vi "ADAM_scan_table.vi"() -> ()   [LabVIEW 2010]
uses:
  Anemometry/Anemometry Sub Vis/Controls/Serveds.ctl
  ADAM Client/Sub VIs/ADAM Controls/Module_type_ADAM.ctl
  ADAM Client/Sub VIs/ADAM Controls/Traverse_Level_State.ctl
  Anemometry/Anemometry Sub Vis/Controls/Post_Process.ctl
  ADAM Client/Sub VIs/ADAM Controls/Channel_State.ctl
  ADAM Client/Sub VIs/ADAM Controls/Ch_description_ADAM.ctl
  ADAM Client/Sub VIs/ADAM Controls/Function_ADAM.ctl
  ADAM Client/Sub VIs/ADAM Controls/Calib_type_ADAM.ctl
  ADAM Client/Sub VIs/ADAM Controls/Address.ctl
  ADAM_Global.vi
  Sub VI's/Channel_Description_Global.vi
  Anemometry/Anemometry Sub Vis/Globals/Meas_global.vi
  Sub VI's/Logged_Data_real_Global.vi
  Anemometry/Anemometry Sub Vis/Globals/Preference_global.vi
  Anemometry/Anemometry Sub Vis/Globals/Gas_management_global.vi
  Anemometry/Anemometry Sub Vis/Globals/Constants_global.vi
panel:
  in  "Reconfigure Gills":bool
  in  "Full Res Pathname":path
  in  "Log full Res Data":bool
  out "Duty No":u16 format="%.0b"
  in  "Save Current setup":bool=TRUE
  in  "Load setup from file":bool
  out "ADAM scan comments":string
  out "History length":i32=250
  in  "stop":bool
  out "Results":dbl[](array[numeric]) format="%.3f"
  out "Titles":string[](array[string])
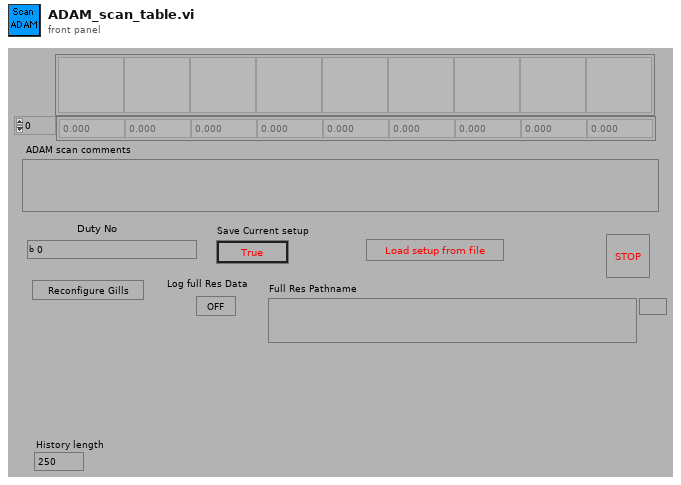
[diagram p1: front panel]
types:
  T1 = enum16{"Load ADAM setup from excel file", "Save ADAM setup to excel file"}
  T2 = typedef "Serveds.ctl" = enum16{"Read Global", "Load Global From File"}
  T3 = typedef "Module_type_ADAM.ctl" = enum16{"4011", "4012", "4013", "4014", "4016", "4017", "4018", "4021", "4050", "4052", "4053", "4060", "4080", "5000", "5017", "5018", "5024", "5051", "5056", "5060", "6060", "Tracker", "WEST", "GILL", "JEM", "VICI", "Vaisala", "DRUCK", "Run VI Named:", "IR2100", "PPT", "Comparator", "VIRTUAL", "Hold Value", "Read A", "Read Ch", "Coded", "Client Info", "Web Client", "X10", "Test"}
  T4 = typedef "Traverse_Level_State.ctl" = enum16{"Running", "Complete"}
  T5 = typedef "Post_Process.ctl" = enum16{"Take New Data", "Post Process Raw Data File"}
  T6 = typedef "Channel_State.ctl" = enum16{"On", "Off", "Always On", "Always Off"}
  T7 = enum16{"Append to Global", "Read Global then Clear"}
  T8 = typedef "Ch_description_ADAM.ctl" = cluster{"Ch Name":string, "Type":T3, "Function":T9, "Ch State":T6, "Calibration type":T10, "A":dbl, "B":dbl, "C":dbl, "D":dbl, "Comments":string, "Address":T11, "String":string, "Duty":u16}
  T9 = typedef "Function_ADAM.ctl" = enum16{"Analogue Input", "Digital Input", "Event counter", "Event rate", "Analogue Output", "Digital Output", "Relay Output"}
  T10 = typedef "Calib_type_ADAM.ctl" = enum16{"Raw", "Bx + A", "Cx^2 + Bx + A", "Dx^3 + Cx^2 + Bx + A", "In Band", "Hi-Tec Q", "Hi-Tec M_dot", "Text"}
  T11 = typedef "Address.ctl" = cluster{"Main":i32, "Ch.":i32, "Sub":i32, "Port Name":string}
  T12 = typedef "Client_State_Cluster.ctl" = cluster{"Client Name":string, "Traverse level State":T4, "People to Email":string[], "Next Contact Time":dbl}
  T13 = typedef "Update_scan_value.ctl" = cluster{"Channel Name":string, "New Value":dbl}
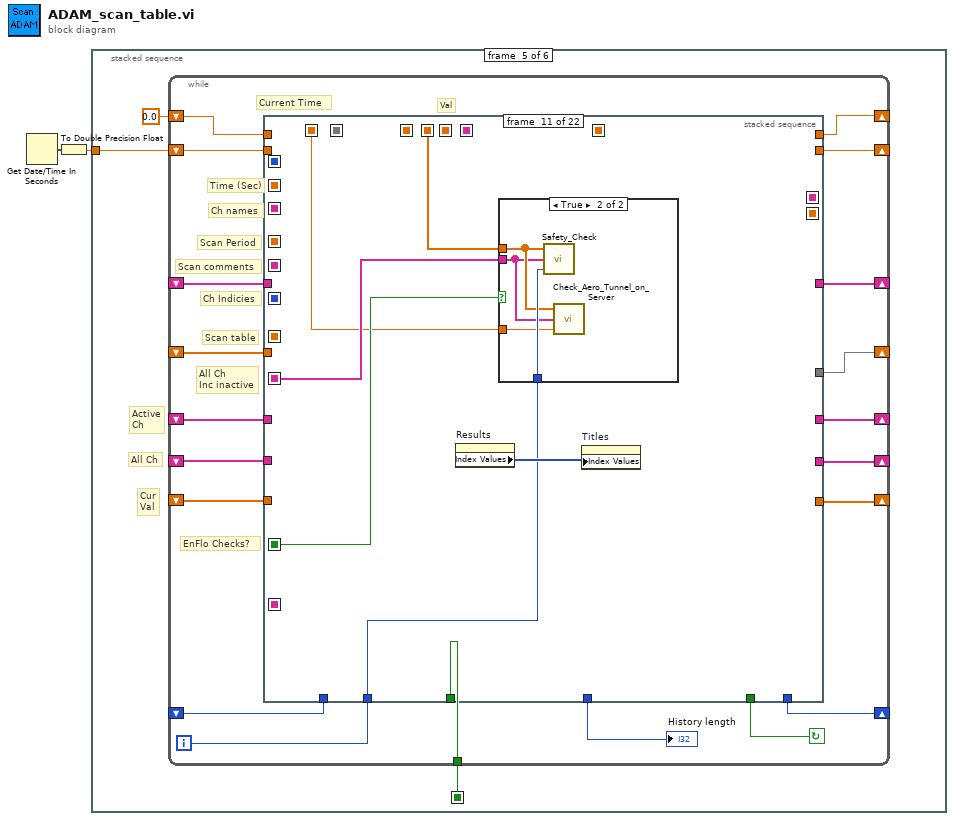
[diagram p0: block diagram]
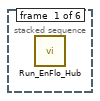
[diagram p2: hidden frame]
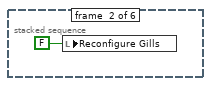
[diagram p3: hidden frame]
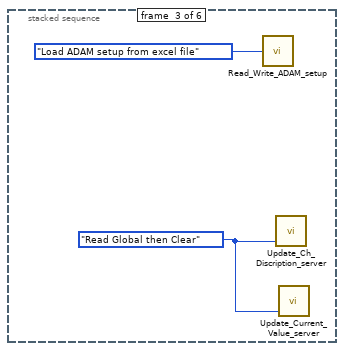
[diagram p4: hidden frame]
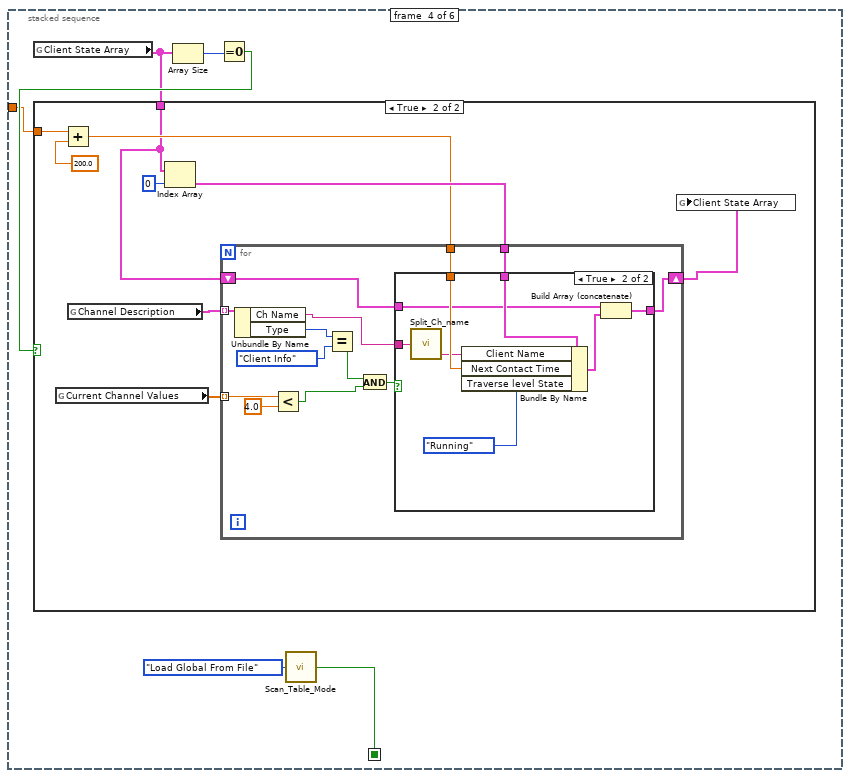
[diagram p5: hidden frame]
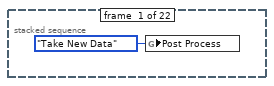
[diagram p8: hidden frame]
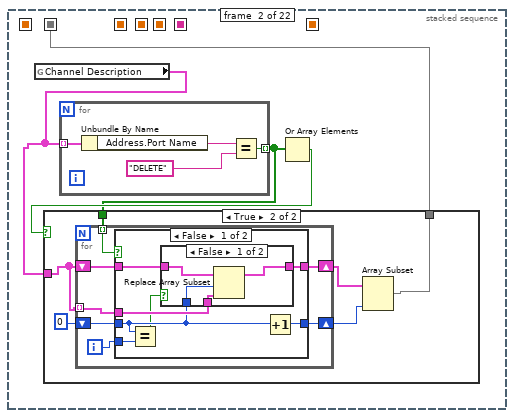
[diagram p9: hidden frame]
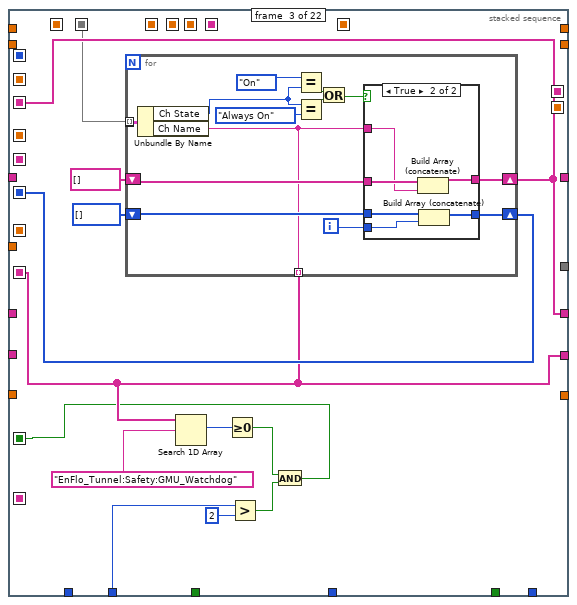
[diagram p13: hidden frame]
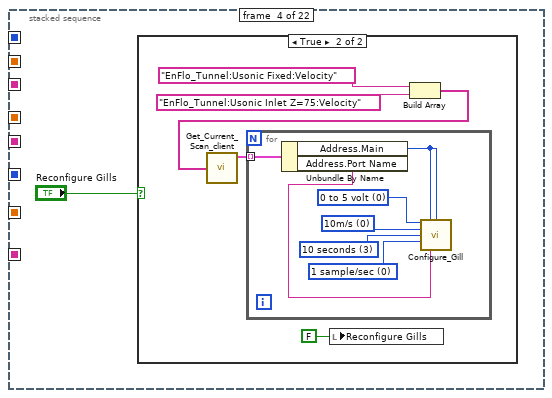
[diagram p15: hidden frame]
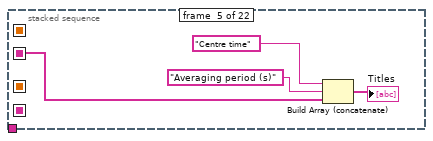
[diagram p17: hidden frame]
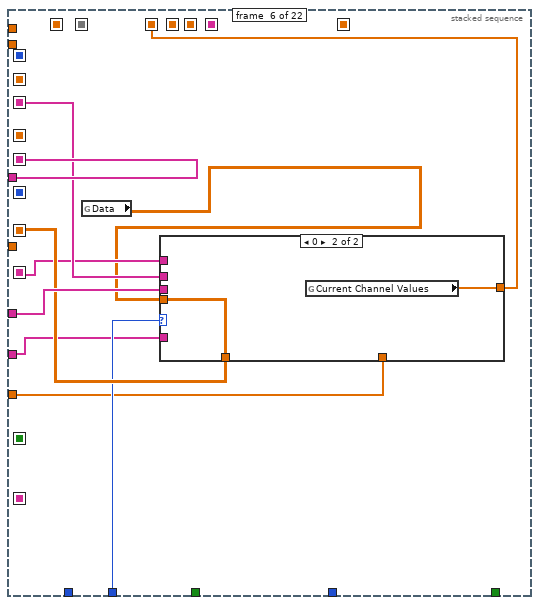
[diagram p18: hidden frame]
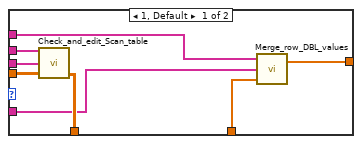
[diagram p19: hidden frame]
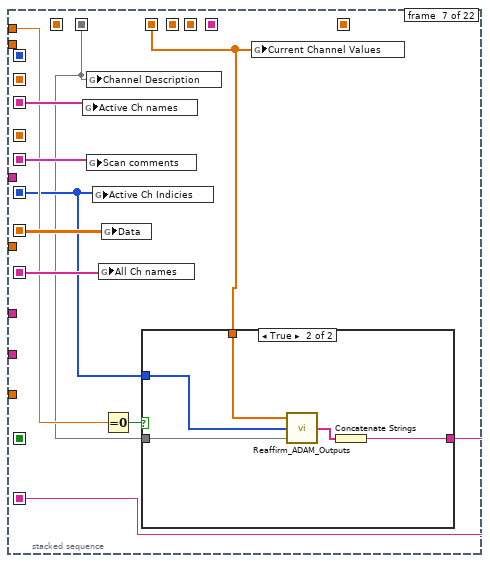
[diagram p20: hidden frame]
diagram:
  n1 = Get Date/Time In Seconds() -> (seconds since 1Jan1904=w2:timestamp)
  n2 = To Double Precision Float(number=w2) -> (double precision float=w1:dbl)
  n3 = stacked-sequence {
    seq-local: [_ _ _ w11 _ _] -> [_ _ _ _ w45 _]
    tunnel: w1 -> [_ _ _ w6 w43 _]
    frame #0 {
      n4 = call "Run_EnFlo_Hub.vi"() -> ()  [unwired: 8 out]
    }
    frame #1 {
      n5 = local write "Reconfigure Gills"(FALSE ("Reconfigure Gills")) -> ()
    }
    frame #2 {
      w4 = T7."Read Global then Clear" ("Mode")
      n6 = call "Read_Write_ADAM_setup.vi"("Mode"=T1."Load ADAM setup from excel file") -> ()  [unwired: 4 out]
      n7 = call "Update_Ch_Discription_server.vi"("Mode"=w4) -> ()  [unwired: 2 in, 1 out]
      n8 = call "Update_Current_Value_server.vi"("Mode"=w4) -> ()  [unwired: 2 in, 1 out]
    }
    frame #3 {
      n9 = global read "ADAM_Global.vi" "Client State Array"() -> (w7:T12[])
      n10 = Array Size(array=w7) -> (size(s)=w9:i32)
      n11 = Equal To 0?(x=w9) -> (x = 0?=w8:bool)
      n12 = case shown="True" w8 {
        tunnel: w7 -> [_ w13]
        tunnel: w6 -> [_ w16]
        frame False {
        }
        frame True {
          n13 = global read "ADAM_Global.vi" "Current Channel Values"() -> (w20:dbl[])
          n14 = Add(x=w16, y=200.0) -> (x+y=w14:dbl)
          n15 = global read "Channel_Description_Global.vi" "Channel Description"() -> (w19:T8[])
          n16 = Index Array(array=w13, index=0) -> (element=w17:T12)
          n17 = for {
            tunnel: w19 -> [w33] mode=indexing
            tunnel: w20 -> [w25] mode=indexing
            tunnel: w17 -> [w26]
            tunnel: w14 -> [w24]
            shift-right: [w23] -> w12
            shift-left: w13 -> [w22]
            n18 = Unbundle By Name(w33) -> ("Ch Name"=w21:string, "Type"=w30:T3)
            n19 = Less?(x=w25, y=4.0) -> (x < y?=w28:bool)
            n20 = Equal?(x=w30, y=Module_type_ADAM."Client Info" ("Type")) -> (x = y?=w29:bool)
            n21 = And(x=w29, y=w28) -> (x .and. y?=w27:bool)
            n22 = case shown="True" w27 {
              tunnel: w26 -> [_ w42]
              tunnel: w24 -> [_ w41]
              tunnel: [w34 w39] -> w23
              tunnel: w22 -> [w34 w38]
              tunnel: w21 -> [_ w36]
              frame False {
              }
              frame True {
                n23 = call "Split_Ch_name.vi"("Ch name"=w36) -> ("Low level"=w35:string)  [unwired: 2 out]
                n24 = Bundle By Name(cluster=w42, "Client Name"=w35, "Next Contact Time"=w41, "Traverse level State"=Traverse_Level_State."Running") -> (w37:T12)
                n25 = Build Array (concatenate)(w38, w37) -> (w39:T12[])
              }
            }
          }
          n26 = global write "ADAM_Global.vi" "Client State Array"(w12) -> ()
        }
      }
      n27 = call "Scan_Table_Mode.vi"("Mode"=Serveds."Load Global From File") -> ("Simulate Mode ?"=w11:bool)
    }
    frame #4 {
      # "Active\nCh"
      # "Cur\nVal"
      # "All Ch"
      n28 = while {
        shift-left: _ -> [w47]
        shift-right: [w46] -> _
        shift-left: _ -> [w48]
        shift-right: [w49] -> _
        shift-left: _ -> [w50]
        shift-right: [w51] -> _
        tunnel: w45 -> [w53]
        shift-left: _ -> [w56]
        shift-right: [w55] -> _
        shift-left: 0.0 -> [w57]
        shift-right: [w52] -> _
        shift-left: _ -> [w59]
        shift-right: [w60] -> _
        shift-left: _ -> [w61]
        shift-right: [w62] -> _
        shift-left: w43 -> [w63]
        shift-right: [w64] -> _
        i -> [w58]
        stop <- w65 continue-if-true
        # "Current Time"
        # "EnFlo Checks?"
        # "Val"
        # "All Ch\nInc inactive"
        # "Scan comments"
        # "Scan table"
        # "Time (Sec)"
        # "Ch Indicies"
        # "Ch names"
        # "Scan Period"
        n29 = stacked-sequence {
          seq-local: [_ _ _ _ _ _ _ _ _ _ _ _ w282 _ _ _ _ _ _ _ _ _] -> [_ _ _ _ _ _ _ _ _ _ _ _ _ _ w333 w338 _ _ _ _ w416 _]
          seq-local: [_ _ _ _ _ _ _ w193 _ _ _ _ _ _ _ _ _ _ _ _ _ _] -> [_ _ _ _ _ _ _ _ _ _ _ _ _ _ _ w345 _ _ _ _ _ _]
          seq-local: [_ _ _ _ _ w160 _ _ _ _ _ _ _ _ _ _ _ _ _ _ _ _] -> [_ _ _ _ _ _ w180 _ _ _ _ _ _ _ _ w343 _ _ _ _ _ _]
          seq-local: [_ _ _ _ _ _ _ w197 _ _ _ _ _ _ _ _ _ _ _ _ _ _] -> [_ _ _ _ _ _ _ _ _ w220 _ w249 _ _ _ w344 _ _ _ _ _ _]
          seq-local: [_ _ _ _ _ w163 _ _ _ _ _ _ _ _ _ _ _ _ _ _ _ _] -> [_ _ _ _ _ _ w182 _ _ _ _ _ _ _ _ _ _ w383 _ _ _ _]
          seq-local: [_ _ _ _ _ _ _ _ _ w218 _ _ _ _ _ _ _ _ _ _ _ _] -> [_ _ _ _ _ _ _ _ _ _ _ _ _ _ _ _ _ w371 _ _ _ _]
          seq-local: [_ _ w114 _ _ _ _ _ _ _ _ _ _ _ _ _ _ _ _ _ _ _] -> [_ _ _ _ w152 w162 w183 w198 _ _ _ _ _ _ _ w341 w346 _ _ _ _ _]
          seq-local: [_ _ w113 _ _ _ _ _ _ _ _ _ _ _ _ _ _ _ _ _ _ _] -> [_ _ _ _ _ _ w176 _ _ w219 _ _ _ _ _ _ _ _ _ _ _ _]
          seq-local: [_ _ _ _ _ w156 _ _ _ _ _ _ _ _ _ _ _ _ _ _ _ _] -> [_ _ _ _ _ _ w177 _ _ w216 _ _ _ _ _ _ _ _ _ _ _ _]
          seq-local: [_ _ _ _ _ _ _ _ _ w214 _ _ _ _ _ _ _ _ _ _ _ _] -> [_ _ _ _ _ _ _ _ _ _ w240 w248 w280 _ _ _ _ _ _ _ _ _]
          seq-local: [_ _ w109 _ _ _ _ _ _ _ _ _ _ _ _ _ _ _ _ _ _ _] -> [_ _ _ _ _ w158 w181 _ _ w215 w239 w247 w281 w306 w325 w340 _ _ _ w393 _ _]
          seq-local: [_ _ _ _ _ _ _ _ w200 _ _ _ _ _ _ _ _ _ _ _ _ _] -> [_ _ _ _ _ _ _ _ _ w213 _ _ _ _ _ _ _ _ _ _ _ _]
          seq-local: [_ w67 _ _ _ _ _ _ _ _ _ _ _ _ _ _ _ _ _ _ _ _] -> [_ _ w111 _ _ _ w175 _ _ w212 _ _ _ _ _ _ _ _ _ _ _ _]
          seq-local: [_ _ _ _ _ _ _ w192 _ _ _ _ _ _ _ _ _ _ _ _ _ _] -> [_ _ _ _ _ _ _ _ _ _ w236 _ _ _ _ _ w348 _ _ _ _ _]
          seq-local: [_ _ _ _ _ _ _ _ _ _ _ _ _ _ _ w337 _ _ _ _ _ _] -> [_ _ _ _ _ _ _ _ _ _ _ _ _ _ _ _ w347 _ _ _ _ _]
          seq-local: [_ _ w103 _ _ _ _ _ _ _ _ _ _ _ _ _ _ _ _ _ _ _] -> [_ _ _ _ _ _ _ w190 _ _ w238 w246 _ _ _ _ _ _ _ _ _ _]
          seq-local: [_ _ _ _ _ _ _ _ _ _ _ _ w279 _ _ _ _ _ _ _ _ _] -> [_ _ _ _ _ _ _ _ _ _ _ _ _ w307 _ _ _ _ _ _ _ _]
          seq-local: [_ _ _ _ _ _ w174 _ _ _ _ _ _ _ _ _ _ _ _ _ _ _] -> [_ _ _ _ _ _ _ _ _ w211 _ _ _ _ _ _ _ _ _ _ _ _]
          seq-local: [_ _ _ _ _ _ _ _ _ _ _ _ w278 _ _ _ _ _ _ _ _ _] -> [_ _ _ _ _ _ _ _ _ _ _ _ _ w305 _ _ _ _ _ _ _ _]
          tunnel: [_ _ _ _ _ _ _ _ _ _ _ _ _ _ _ _ _ _ w391 _ _ _] -> w65
          tunnel: [_ _ _ _ _ _ _ w192 _ _ _ _ _ _ _ _ _ _ _ _ _ _] -> w64
          tunnel: w63 -> [_ _ _ _ _ _ _ w194 _ _ _ _ _ _ _ _ _ _ _ _ _ _]
          tunnel: [_ _ _ _ _ _ _ _ _ _ _ _ _ _ _ _ _ w381 _ _ _ _] -> w62
          tunnel: w61 -> [_ _ _ _ _ w163 _ _ _ _ _ _ _ _ _ _ _ _ _ _ _ _]
          tunnel: [_ _ w114 _ _ _ _ _ _ _ _ _ _ _ _ _ _ _ _ _ _ _] -> w60
          tunnel: w59 -> [_ _ _ _ _ w161 _ _ _ _ _ _ _ w308 _ _ _ _ _ _ _ _]
          tunnel: w58 -> [_ _ w107 _ _ w159 _ _ _ _ w237 _ _ _ _ _ _ _ w389 _ _ w420]
          tunnel: w57 -> [_ _ _ _ _ _ w178 _ _ _ _ w251 _ _ _ _ _ _ _ _ _ _]
          tunnel: [_ _ _ _ _ _ _ _ _ _ _ w253 _ _ _ _ _ _ _ _ _ _] -> w52
          tunnel: w56 -> [_ _ _ _ _ _ _ _ _ _ _ _ _ _ w331 _ _ _ _ _ _ _]
          tunnel: [_ _ _ _ _ _ _ _ _ _ _ _ _ _ w327 _ _ _ _ _ _ _] -> w55
          tunnel: [_ _ _ _ _ _ _ _ _ _ _ _ _ _ _ w342 _ _ _ _ _ _] -> w54
          tunnel: w53 -> [_ _ _ _ _ _ _ _ _ w217 _ _ _ _ _ _ _ _ _ _ _ _]
          tunnel: [_ _ w109 _ _ _ _ _ _ _ _ _ _ _ _ _ _ _ _ _ _ _] -> w51
          tunnel: w50 -> [_ _ _ _ _ w157 _ _ _ _ _ _ _ _ _ _ _ _ _ _ _ _]
          tunnel: [_ _ _ _ _ _ _ _ _ _ _ _ _ _ _ _ _ _ _ _ w416 _] -> w49
          tunnel: w48 -> [_ _ _ _ _ w155 _ _ _ _ _ _ _ _ _ _ _ _ _ _ _ _]
          tunnel: w47 -> [_ _ _ _ _ _ _ _ w201 _ _ _ _ _ _ _ _ _ _ _ _ _]
          tunnel: [_ _ _ _ _ _ _ _ w202 _ _ _ _ _ _ _ _ _ _ _ _ _] -> w46
          frame #0 {
            n30 = global write "Meas_global.vi" "Post Process"(Post_Process."Take New Data" ("Post Process")) -> ()
          }
          frame #1 {
            n31 = global read "Channel_Description_Global.vi" "Channel Description"() -> (w69:T8[])
            n32 = for {
              tunnel: w69 -> [w102] mode=indexing
              tunnel: [w99] -> w68 mode=indexing
              n33 = Unbundle By Name(w102) -> ("Address.Port Name"=w101:string)
              n34 = Equal?(x=w101, y="DELETE") -> (x = y?=w99:bool)
            }
            n35 = Or Array Elements(Boolean array=w68) -> (logical OR=w70:bool)
            n36 = case shown="True" w70 {
              tunnel: w69 -> [w71 w75]
              tunnel: w68 -> [_ w77]
              tunnel: [w71 w72] -> w67
              frame False {
              }
              frame True {
                n37 = for {
                  shift-right: [w84] -> w74
                  shift-left: w75 -> [w83]
                  tunnel: w77 -> [w79] mode=indexing
                  shift-right: [w82] -> w73
                  shift-left: 0 -> [w80]
                  tunnel: w75 -> [w81] mode=indexing
                  i -> [w78]
                  n38 = case shown="False" w79 {
                    tunnel: [w90 w98] -> w84
                    tunnel: w83 -> [w91 w98]
                    tunnel: [w88 w97] -> w82
                    tunnel: w80 -> [w87 w97]
                    tunnel: w81 -> [w89 _]
                    tunnel: w78 -> [w86 _]
                    frame False {
                      n39 = Equal?(x=w87, y=w86) -> (x = y?=w85:bool)
                      n40 = case shown="False" w85 {
                        tunnel: w91 -> [w95 w96]
                        tunnel: [w94 w96] -> w90
                        tunnel: w89 -> [w93 _]
                        tunnel: w87 -> [w92 _]
                        frame False {
                          n41 = Replace Array Subset(array=w95, new element=w93, index=w92) -> (w94:T8[])
                        }
                        frame True {
                        }
                      }
                      n42 = Increment(x=w87) -> (x+1=w88:i32)
                    }
                    frame True {
                    }
                  }
                }
                n43 = Array Subset(array=w74, length=w73) -> (w72:T8[])  [unwired: 1 in]
              }
            }
          }
          frame #2 {
            n44 = for {
              tunnel: [w128] -> _ mode=indexing
              shift-right: [w127] -> w114
              shift-left: string[] [] -> [w118]
              shift-right: [w124] -> w113
              shift-left: i32[] [] -> [w126]
              tunnel: [w116] -> w109 mode=indexing
              tunnel: w111 -> [w128] mode=indexing
              i -> [w125]
              n45 = Unbundle By Name(w128) -> ("Ch State"=w119:T6, "Ch Name"=w116:string)
              n46 = Equal?(x=Channel_State."On" ("Channel State"), y=w119) -> (x = y?=w121:bool)
              n47 = Equal?(x=w119, y=Channel_State."Always On" ("Channel State")) -> (x = y?=w120:bool)
              n48 = Or(x=w121, y=w120) -> (x .or. y?=w117:bool)
              n49 = case shown="True" w117 {
                tunnel: w118 -> [w129 w136]
                tunnel: w116 -> [_ w135]
                tunnel: [w129 w134] -> w127
                tunnel: w126 -> [w130 w133]
                tunnel: w125 -> [_ w132]
                tunnel: [w130 w131] -> w124
                frame False {
                }
                frame True {
                  n50 = Build Array (concatenate)(w136, w135) -> (w134:string[])
                  n51 = Build Array (concatenate)(w133, w132) -> (w131:i32[])
                }
              }
            }
            n52 = Search 1D Array(1D array=w109, element="EnFlo_Tunnel:Safety:GMU_Watchdog") -> (index of element=w108:i32)  [unwired: 1 out]
            n53 = Greater Or Equal To 0?(x=w108) -> (x >= 0?=w104:bool)
            n54 = Greater?(x=w107, y=2) -> (0:w105:bool)
            n55 = And(x=w104, y=w105) -> (x .and. y?=w103:bool)
          }
          frame #3 {
            n56 = case shown="True" "Reconfigure Gills" {
              frame False {
              }
              frame True {
                n57 = local write "Reconfigure Gills"(FALSE ("Reconfigure Gills")) -> ()
                n58 = Build Array("EnFlo_Tunnel:Usonic Fixed:Velocity", "EnFlo_Tunnel:Usonic Inlet Z=75:Velocity") -> (w140:string[])
                n59 = call "Get_Current_Scan_client.vi"("ADAM Ch Names"=w140) -> ("Ch Description Array"=w139:T8[])  [unwired: 3 out]
                n60 = for {
                  tunnel: w139 -> [w145] mode=indexing
                  w149 = u16 0 items=["1 sample/sec", "4 samples/sec"] ("Samples/sec")
                  w148 = u16 3 items=["OFF", "3 seconds", "5 seconds", "10 seconds"] ("Averaging Time")
                  w147 = u16 0 items=["10m/s", "20m/s", "30m/s", "40m/s", "50m/s", "60m/s", "70m/s"] ("Analogue O/P Scale")
                  w146 = u16 0 items=["0 to 5 volt", "+/-2.5 Volt", "4-20mA"] ("Analogue O/P Config")
                  n61 = Unbundle By Name(w145) -> ("Address.Main"=w144:i32, "Address.Port Name"=w143:string)
                  n62 = call "Configure_Gill.vi"("Analogue O/P Config"=w146, "ORIGINAL Address"=w144, "NEW Address"=w144, "Analogue O/P Scale"=w147, "Averaging Time"=w148, "Samples/sec"=w149, "Port Name"=w143) -> ()  [unwired: 9 out]
                }
              }
            }
          }
          frame #4 {
            n63 = Build Array (concatenate)("Centre time", "Averaging period (s)", w152) -> (→"Titles":string[])
          }
          frame #5 {
            n64 = global read "Logged_Data_real_Global.vi" "Data"() -> (w154:dbl[][])
            n65 = case shown="0" w159 {
              tunnel: w154 -> [w171 w173]
              tunnel: w162 -> [w168 _]
              tunnel: w161 -> [w170 _]
              tunnel: [w169 w173] -> w160
              tunnel: w158 -> [w167 _]
              tunnel: w157 -> [w166 _]
              tunnel: [w165 w172] -> w156
              tunnel: w155 -> [w164 _]
              frame 1, Default {
                n66 = call "Check_and_edit_Scan_table.vi"("2D array input"=w171, "Original Channels"=w170, "Present Channels"=w168) -> ("2D array output"=w169:dbl[][])  [unwired: 2 out]
                n67 = call "Merge_row_DBL_values.vi"("Present Row values"=w164, "Present Channels"=w166, "Desired Channels"=w167) -> ("Desired Row values"=w165:dbl[])  [unwired: 1 out]
              }
              frame 0 {
                n68 = global read "ADAM_Global.vi" "Current Channel Values"() -> (w172:dbl[])
              }
            }
          }
          frame #6 {
            n69 = global write "ADAM_Global.vi" "Active Ch names"(w183) -> ()
            n70 = global write "Channel_Description_Global.vi" "Channel Description"(w175) -> ()
            n71 = global write "ADAM_Global.vi" "Scan comments"(w182) -> ()
            n72 = global write "ADAM_Global.vi" "Active Ch Indicies"(w176) -> ()
            n73 = global write "ADAM_Global.vi" "All Ch names"(w181) -> ()
            n74 = global write "Logged_Data_real_Global.vi" "Data"(w180) -> ()
            n75 = Equal To 0?(x=w178) -> (x = 0?=w179:bool)
            n76 = case shown="True" w179 {
              tunnel: w177 -> [_ w189]
              tunnel: w176 -> [_ w188]
              tunnel: w175 -> [_ w187]
              tunnel: ["" w185] -> w174
              frame False {
              }
              frame True {
                n77 = call "Reaffirm_ADAM_Outputs.vi"("Channel Description"=w187, "Active Ch Indicies"=w188, "Current Channel Values"=w189) -> ("Scan Comments"=w186:string[])  [unwired: 2 out]
                n78 = Concatenate Strings(w186) -> (w185:string)
              }
            }
            n79 = global write "ADAM_Global.vi" "Current Channel Values"(w177) -> ()
          }
          frame #7 {
            n80 = case shown="True" w190 {
              tunnel: w198 -> [_ w199]
              frame False {
              }
              frame True {
                n81 = call "Gas_Status_panel.vi"("Ch names"=w199) -> ()  [unwired: 15 out]
              }
            }
            n82 = Get Date/Time In Seconds() -> (seconds since 1Jan1904=w191:timestamp)
            n83 = To Double Precision Float(number=w191) -> (double precision float=w192:dbl)
            n84 = Subtract(x=w192, y=w194) -> (x-y=w197:dbl)
            n85 = Divide(x=w197, y=2.0) -> (x/y=w195:dbl)
            n86 = Add(x=w195, y=w194) -> (x+y=w193:dbl)
          }
          frame #8 {
            n87 = Equal To 0?(x=w201) -> (x = 0?=w205:bool)
            n88 = Equal?(x=u16 32768, y=w201) -> (x = y?=w204:bool)
            n89 = Select(t=u16 1, s=w205, f=w201) -> (s? t:f=w200:u16)
            "Duty No" <- w200
            n90 = case shown="False" w204 {
              tunnel: [w207 u16 0] -> w202
              tunnel: w200 -> [w209 _]
              frame False {
                n91 = Multiply(x=u16 2, y=w209) -> (x*y=w207:u16)
              }
              frame True {
              }
            }
          }
          frame #9 {
            n92 = for {
              tunnel: w212 -> [w227]
              tunnel: w220 -> [w235]
              shift-right: [w233] -> w214
              shift-left: w216 -> [w231]
              tunnel: w215 -> [w232]
              shift-right: [w228] -> w218
              shift-left: w211 -> [w230]
              tunnel: w219 -> [w222] mode=indexing
              tunnel: w216 -> [w224]
              tunnel: w217 -> [w225]
              tunnel: w213 -> [w221]
              n93 = Index Array(array=w224, index=w222) -> (element=w223:dbl)
              n94 = Index Array(array=w227, index=w222) -> (element=w226:T8)
              n95 = call "Adam_Ch_Input_Output.vi"("Simulate"=w225, "Duty No"=w221, "Previuos Scan Value"=w223, "Ch values"=w231, "Scan Period"=w235, "Ch Discription"=w226, "Ch names"=w232) -> ("Scan comment"=w229:string, "Calibrated units"=w234:dbl)  [unwired: 1 in, 2 out]
              n96 = Concatenate Strings(w230, w229) -> (w228:string)
              n97 = Replace Array Subset(array=w231, new element=w234, index=w222) -> (w233:dbl[])
            }
          }
          frame #10 {
            n98 = property on="Results" class="Arr (strict)"() -> ("Index Values"=w241:u32[])  [unwired: 2 in, 2 out]
            n99 = case shown="True" w238 {
              tunnel: w240 -> [_ w244]
              tunnel: w239 -> [_ w243]
              tunnel: w237 -> [_ w245]
              tunnel: w236 -> [_ w242]
              frame False {
              }
              frame True {
                n100 = call "Safety_Check.vi"("Adam Loop Count"=w245, "Ch Names"=w243, "Values"=w244) -> ()  [unwired: 1 out]
                n101 = call "Check_Aero_Tunnel_on_Server.vi"("Current Time"=w242, "Ch Names"=w243, "Values"=w244) -> ()  [unwired: 1 in]
              }
            }
            n102 = property on="Titles" class="Arr (strict)"("Index Values"=w241) -> ()  [unwired: 2 in, 2 out]
          }
          frame #11 {
            n103 = Greater?(x=w251, y=60.0) -> (0:w252:bool)
            n104 = case shown="True" w252 {
              tunnel: [w255 w260] -> w253
              tunnel: w251 -> [w256 _]
              tunnel: w249 -> [w254 _]
              tunnel: w248 -> [_ w259]
              tunnel: w247 -> [_ w258]
              tunnel: w246 -> [_ w257]
              frame False {
                n105 = Add(x=w256, y=w254) -> (x+y=w255:dbl)
              }
              frame True {
                n106 = stacked-sequence {
                  tunnel: [0.0 _] -> w260
                  tunnel: w259 -> [_ w275]
                  tunnel: w258 -> [_ w274]
                  tunnel: w257 -> [_ w273]
                  frame #0 {
                    n107 = case shown="False" "Save Current setup" {
                      tunnel: [FALSE w265] -> w261
                      frame False {
                      }
                      frame True {
                        n108 = Get Date/Time In Seconds() -> (seconds since 1Jan1904=w267:timestamp)
                        n109 = global read "ADAM_Global.vi" "Network Last checked"() -> (w271:dbl)
                        n110 = To Double Precision Float(number=w267) -> (double precision float=w266:dbl)
                        n111 = Subtract(x=w271, y=w266) -> (x-y=w270:dbl)
                        n112 = Absolute Value(x=w270) -> (abs(x)=w269:dbl)
                        n113 = Less?(x=w269, y=1.5) -> (x < y?=w265:bool)
                      }
                    }
                    n114 = case shown="True" w261 {
                      frame False {
                      }
                      frame True {
                        n115 = call "Read_Write_ADAM_setup.vi"("Mode"=T1."Save ADAM setup to excel file") -> ()  [unwired: 4 out]
                      }
                    }
                  }
                  frame #1 {
                    n116 = case shown="True" w273 {
                      tunnel: w275 -> [_ w277]
                      tunnel: w274 -> [_ w276]
                      frame False {
                      }
                      frame True {
                        n117 = call "Do_Every_minute.vi"("Ch Names"=w276, "Values"=w277) -> ()  [unwired: 1 out]
                      }
                    }
                  }
                }
              }
            }
          }
          frame #12 {
            n118 = call "Update_Current_Value_server.vi"("Mode"=T7."Read Global then Clear") -> ("Update array out"=w284:T13[])  [unwired: 2 in]
            n119 = for {
              tunnel: w281 -> [w292]
              tunnel: w284 -> [w287] mode=indexing
              shift-right: [w290] -> w282
              shift-left: w280 -> [w291]
              tunnel: [w286] -> w279 mode=indexing
              tunnel: [w285] -> w278 mode=indexing
              n120 = Unbundle By Name(w287) -> ("Channel Name"=w286:string, "New Value"=w285:dbl)
              n121 = Search 1D Array(1D array=w292, element=w286) -> (index of element=w289:i32)  [unwired: 1 out]
              n122 = Less Than 0?(x=w289) -> (x < 0?=w288:bool)
              n123 = case shown="True" w288 {
                tunnel: w286 -> [_ w293]
                tunnel: w287 -> [_ w298]
                frame False {
                }
                frame True {
                  n124 = global read "ADAM_Global.vi" "Update Current Value"() -> (w297:T13[])
                  n125 = call "Check_Ch_Name_colons.vi"("No of Colons"=2, "Ch Name in"=w293) -> ("Ch Name out"=w294:string)
                  n126 = Bundle By Name(cluster=T8 {"Ch Name"="", "Type"=enum."Hold Value", "Function"=enum."Analogue Input", "Ch State"=enum."On", "Calibration type"=enum."Raw", "A"=0.0, "B"=0.0, "C"=0.0, "D"=0.0, "Comments"="", "Address"={"Main"=0, "Ch."=0, "Sub"=0, "Port Name"=""}, "String"="", "Duty"=65535} ("Ch Description"), "Ch Name"=w294, "Type"=Module_type_ADAM."Hold Value") -> (w302:T8)
                  n127 = Build Array (concatenate)(w297, w298) -> (w296:T13[])
                  n128 = global write "ADAM_Global.vi" "Update Current Value"(w296) -> ()
                  n129 = global read "Preference_global.vi" "Rig Setup"() -> (w300:string)
                  n130 = Build Array(w302) -> (w301:T8[])
                  n131 = call "Update_Ch_Discription_server.vi"("Mode"=T7."Append to Global", "Client HD name"=w300, "Channels to update In"=w301) -> ()  [unwired: 1 out]
                }
              }
              n132 = Replace Array Subset(array=w291, new element=w285, index=w289) -> (w290:dbl[])
            }
          }
          frame #13 {
            n133 = for {
              tunnel: w308 -> [w316]
              tunnel: w307 -> [w314] mode=indexing
              tunnel: w306 -> [w315]
              tunnel: w305 -> [w312] mode=indexing
              n134 = Search 1D Array(1D array=w316, element=w314) -> (index of element=w313:i32)  [unwired: 1 out]
              n135 = Less Than 0?(x=w313) -> (x < 0?=w311:bool)
              n136 = Not Equal To 0?(x=w312) -> (x != 0?=w310:bool)
              n137 = And(x=w310, y=w311) -> (x .and. y?=w309:bool)
              n138 = case shown="True" w309 {
                tunnel: w315 -> [_ w324]
                tunnel: w314 -> [_ w323]
                frame False {
                }
                frame True {
                  n139 = Search 1D Array(1D array=w324, element=w323) -> (index of element=w318:i32)  [unwired: 1 out]
                  n140 = global read "Channel_Description_Global.vi" "Channel Description"() -> (w319:T8[])
                  n141 = Index Array(array=w319, index=w318) -> (element=w322:T8)
                  n142 = Bundle By Name(cluster=w322, "Ch State"=Channel_State."On") -> (w320:T8)
                  n143 = Replace Array Subset(array=w319, new element=w320, index=w318) -> (w317:T8[])
                  n144 = global write "Channel_Description_Global.vi" "Channel Description"(w317) -> ()
                }
              }
            }
          }
          frame #14 {
            n145 = Search 1D Array(1D array=w325, element="GMU:Source:Release Temp") -> (index of element=w332:i32)  [unwired: 1 out]
            n146 = Index Array(array=w333, index=w332) -> (element=w330:dbl)
            n147 = Build Array (concatenate)(w330, w331) -> (w329:dbl[])
            n148 = Array Subset(array=w329, length=10 ("Array Length")) -> (w327:dbl[])  [unwired: 1 in]
            n149 = call "Mean_fr_NaN_data.vi"("Data"=w327) -> ("Mean value"=w326:dbl)
            n150 = global write "Gas_management_global.vi" "Release temp (deg C)"(w326) -> ()
          }
          frame #15 {
            w335 = 250000  # Table size
            n151 = call "Merge_row_DBL_values.vi"("Present Row values"=w338, "Present Channels"=w340, "Desired Channels"=w341) -> ("Desired Row values"=w339:dbl[])  [unwired: 1 out]
            n152 = Build Array (concatenate)(w345, w344, w339) -> (w337:dbl[])
            "Results" <- w337
            n153 = call "Manipulate_Table.vi"("Table size"=w335, "Latest Row"=w337, "Table Input"=w343) -> ("History length"=w342:i32, "Table Output"=w336:dbl[][])  [unwired: 1 out]
            n154 = global write "Logged_Data_real_Global.vi" "Data"(w336) -> ()
          }
          frame #16 {
            n155 = case shown="True" "Log full Res Data" {
              tunnel: w348 -> [_ w361]
              tunnel: w347 -> [_ w360]
              tunnel: w346 -> [_ w359]
              frame False {
              }
              frame True {
                n156 = Build Array (concatenate)(w361, w360) -> (w358:dbl[])
                n157 = Number To Fractional String(number=w358) -> (F-format string=w356:string[])  [unwired: 3 out]
                n158 = call "Does_file_exist_(simple).vi"("Pathname"="Full Res Pathname") -> ("exists?"=w355:bool)
                n159 = Build Array (concatenate)("Current time", "Centre Time", "Averaging period (s)", w359) -> (w357:string[])
                n160 = case shown="False" w355 {
                  tunnel: w357 -> [w367 _]
                  tunnel: w356 -> [w366 w368]
                  tunnel: [w363 w369] -> w351
                  frame False {
                    n161 = Build Array(w367, w366) -> (w364:string[][])
                    n162 = Array To Spreadsheet String(array=w364, 3:"%s" ("format string")) -> (spreadsheet string=w363:string)  [unwired: 1 out]
                  }
                  frame True {
                    n163 = Array To Spreadsheet String(array=w368, 3:"%s" ("format string")) -> (spreadsheet string=w369:string)  [unwired: 1 out]
                  }
                }
                n164 = call "Write_File_Simple.vi"("append to file? (new file:F)"=TRUE, "character string"=w351, "file path"="Full Res Pathname") -> ()  [unwired: 2 out]
              }
            }
          }
          frame #17 {
            w379 = 150 ("length")
            w380 = 50  # History length
            n165 = String Subset(string=w371, length (rest)=w379) -> (substring=w373:string)  [unwired: 1 out]
            n166 = String Length(string=w373) -> (length=w378:i32)
            n167 = Equal?(x=w379, y=w378) -> (x = y?=w377:bool)
            n168 = Select(t=" Clipped ", s=w377, f="") -> (s? t:f=w374:string)
            n169 = Concatenate Strings(w374, w373) -> (w372:string)
            n170 = Build Array (concatenate)(w383, w372) -> (w382:string[])
            n171 = Array Size(array=w382) -> (size(s)=w385:i32)
            n172 = Subtract(x=w385, y=w380) -> (x-y=w384:i32)
            n173 = Array Subset(array=w382, index=w384) -> (w381:string[])  [unwired: 1 in]
            "ADAM scan comments" <- w371
          }
          frame #18 {
            n174 = Format Into String(format string="%s %d %s" ("Format String"), "\nScan No " ("Header message"), w389, "\r") -> (resulting string=w388:string)  [unwired: 2 in, 1 out]
            n175 = call "Write_out_serial_log.vi"("Header message"=w388) -> ()
            n176 = Not(x="stop") -> (.not. x?=w391:bool)
          }
          frame #19 {
            n177 = call "Update_Ch_Discription_server.vi"("Mode"=T7."Read Global then Clear") -> ("Channels to update Out"=w394:T8[])  [unwired: 2 in]
            n178 = Array Size(array=w394) -> (size(s)=w396:i32)
            n179 = Equal To 0?(x=w396) -> (x = 0?=w395:bool)
            n180 = case shown="False" w395 {
              tunnel: w393 -> [w401 _]
              tunnel: w394 -> [w400 _]
              frame False {
                n181 = global read "Channel_Description_Global.vi" "Channel Description"() -> (w399:T8[])
                n182 = for {
                  tunnel: w401 -> [w408]
                  tunnel: w400 -> [w405] mode=indexing
                  shift-right: [w404] -> w398
                  shift-left: w399 -> [w407]
                  n183 = Unbundle By Name(w405) -> ("Ch Name"=w406:string)
                  n184 = Search 1D Array(1D array=w408, element=w406) -> (index of element=w402:i32)  [unwired: 1 out]
                  n185 = Less Than 0?(x=w402) -> (x < 0?=w403:bool)
                  n186 = case shown="False" w403 {
                    tunnel: w407 -> [w412 w415]
                    tunnel: w405 -> [w411 w413]
                    tunnel: [w410 w414] -> w404
                    tunnel: w402 -> [w409 _]
                    frame False {
                      n187 = Replace Array Subset(array=w412, new element=w411, index=w409) -> (w410:T8[])
                    }
                    frame True {
                      n188 = Build Array (concatenate)(w415, w413) -> (w414:T8[])
                    }
                  }
                }
                n189 = global write "Channel_Description_Global.vi" "Channel Description"(w398) -> ()
              }
              frame True {
              }
            }
          }
          frame #20 {
            n190 = case shown="True" "Load setup from file" {
              frame False {
              }
              frame True {
                n191 = local write "Save Current setup"(TRUE ("Save Current setup")) -> ()
                n192 = call "Read_Write_ADAM_setup.vi"("Mode"=T1."Load ADAM setup from excel file") -> ()  [unwired: 4 out]
              }
            }
          }
          frame #21 {
            n193 = case shown="0" w420 {
              frame 0 {
                w424 = path "ADAM Server/Log_ADAM_scan_table.vi"  # :ADAM Server:Log_ADAM_scan_table.vi
                n194 = global read "Constants_global.vi" "EnFlo SW Folder"() -> (w425:path)
                n195 = Build Path(base path=w425, name or relative path=path "ADAM Client/ADAM client VIs/Plot_Server_Data.vi") -> (appended path=w422:path)
                n196 = Build Path(base path=w425, name or relative path=w424) -> (appended path=w423:path)
                n197 = Build Array(w423, w422) -> (w421:path[])
                n198 = for {
                  tunnel: w421 -> [w427] mode=indexing
                  n199 = Open VI Reference(vi path=w427) -> (vi reference=w431:refnum<vi>, error out=w430:errorcluster)  [unwired: 2 in, 3 out]
                  n200 = property class="VI"(reference=w431, error in=w430, "Front Panel Window:Open"=TRUE) -> (reference out=w428:refnum<vi>, error out=w429:errorcluster)
                  n201 = invoke class="VI" method="Run VI"(reference=w428, error in=w429, "Wait until done"=FALSE) -> (reference out=w435:refnum<vi>, error out=w434:errorcluster)  [unwired: 2 in, 3 out]
                  n202 = Close Reference(reference=w435, error in (no error)=w434) -> ()  [unwired: 1 out]
                }
              }
              frame 1, Default {
              }
            }
          }
        }
        "History length" <- w54
      }
    }
    frame #5 {
      n203 = call "Read_Write_ADAM_setup.vi"("Mode"=T1."Save ADAM setup to excel file") -> ()  [unwired: 4 out]
    }
  }
